vi "Get Sample Clock Rate.vi"(0 "device session in":refnum<class "Device Session.lvclass">, 11 "error in":errorcluster) -> (4 "device session out":refnum<class "Device Session.lvclass">, 6 "sample clock rate (Hz)":dbl, 15 "error out":errorcluster)   [LabVIEW 2021, in "Device Session.lvclass"]
doc: "Returns the sample rate of the configured clock.\n\n<B>Input Parameters</B>\n\n<B>device session in</B> is a reference to the Device Session object, which contains a session to each instrument design library used in this sample project. This parameter is obtained from the 'Open Session' VI.\n\n<B>error in</B> describes error conditions that occur before this node runs. This input provides standard 'error in' functionality.\n\n<B>Output Parameters</B>\n\n<B>device session out</B> passes a reference to the session to the next VI.\n\n<B>sample clock rate (Hz)</B> is the sample rate of the configured clock.\n\n<B>error out</B> contains error information. This output provides standard 'error out' functionality."
uses:
  Device Session.lvclass
  Device Session.lvclass/Device Session.ctl
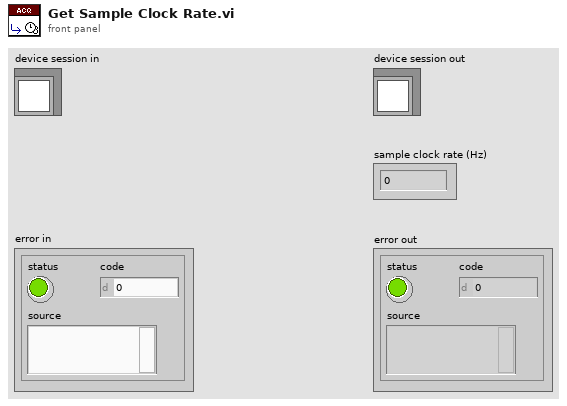
[diagram p1: front panel]
types:
  T1 = typedef "Device Session.lvclass/Device Session Object.ctl" = cluster{"fpga reference":T2, "reg bus":refnum<class "niInstr FIFO Register Bus v1 Host.lvclass">, "subsystem map":refnum<class "niInstr Subsystem Map v1 Host.lvclass">, "cal data":refnum<class "niHSAI Cal Data v1 Host.lvclass">, "config":refnum<class "niHSAI Group A Config v1 Host.lvclass">, "acquisition 0":refnum<class "niInstr Multirecord Acquisition v1 Host.lvclass">, "acquisition 1":refnum<class "niInstr Multirecord Acquisition v1 Host.lvclass">, "number of selected acq channels":u8, "selected acq channels":bool[], "number of channels":u32, "configured channels":bool[], "acq configuration":cluster{"number of samples":u64, "number of records":u64, "pretrigger samples":u64}, "actual channel configuration":T3[], "sample clock rate (Hz)":dbl, "scaling coefficients":T7[]}
  T2 = typedef "Device Session.lvclass/FPGA Refnum.ctl" = refnum<k20>
  T3 = typedef "niHSAI Types v1 Host.lvlib/Channel Configuration.ctl" = cluster{"channel":u32, "coupling":T4, "impedance":T5, "bandwidth":T6, "vertical range":dbl, "vertical offset":dbl}
  T4 = typedef "niHSAI Types v1 Host.lvlib/Coupling.ctl" = enum8{"Default", "DC", "AC"}
  T5 = typedef "niHSAI Types v1 Host.lvlib/Impedance.ctl" = enum8{"Default", "1 mega ohm", "50 ohm"}
  T6 = typedef "niHSAI Types v1 Host.lvlib/Bandwidth.ctl" = enum8{"Default", "Full Bandwidth", "Anti-alias Filter", "150 MHz"}
  T7 = typedef "niInstr Multirecord Acquisition v1 Host.lvclass/Scaling Coefficient.ctl" = cluster{"gain":dbl, "offset":dbl}
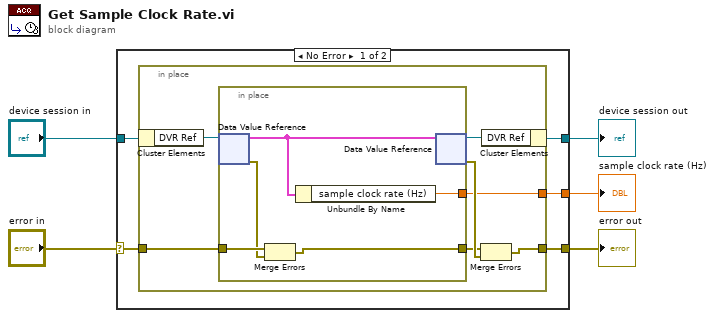
[diagram p0: block diagram]
diagram:
  n1 = case shown="No Error" "error in" {
    selector: "error in" -> [w10 w24]
    tunnel: [w8 w24] -> w4
    tunnel: "device session in" -> [w7 w23]
    tunnel: [w6 w23] -> w2
    tunnel: [w9 _] -> w1
    frame No Error {
      n2 = in-place {
        in-place-border: w10 -> [w17]
        in-place-border: [w15] -> w9
        in-place-border: [w11] -> w8
        n3 = in-place-cluster #1(w7) -> ("DVR Ref"=w13:refnum<data-value>)
        n4 = in-place {
          in-place-border: w17 -> [w22]
          in-place-border: [w19] -> w15
          in-place-border: [w18] -> w14
          n5 = in-place-dvr #2(w13) -> (w20:T1, w21:errorcluster)
          n6 = Merge Errors(w22, w21) -> (w18:errorcluster)
          n7 = Unbundle By Name(w20) -> ("sample clock rate (Hz)"=w19:dbl)
          n8 = in-place-dvr #2(w20) -> (w12:refnum<data-value>, w16:errorcluster)
        }
        n9 = Merge Errors(w14, w16) -> (w11:errorcluster)
        n10 = in-place-cluster #1("DVR Ref"=w12) -> (w6:refnum<class "Device Session.lvclass">)
      }
    }
    frame Error {
    }
  }
  "error out" <- w4
  "device session out" <- w2
  "sample clock rate (Hz)" <- w1
